vi "Update Front Panel.vi"() -> (3 "Battlefield":i32[][](array[numeric]))   [LabVIEW 2015, in "SB SubVIs.lvlib"]
uses:
  SB SubVIs.lvlib
  Globals.vi
  Globals (private).vi
  Square/Square.lvclass
  Endigit Library/Endigit.lvlib
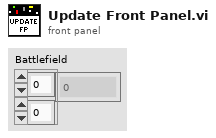
[diagram p1: front panel]
types:
  T1 = typedef "SB Type Defs.lvlib/Square Cluster.ctl" = cluster{"Attacked":bool, "Team":i32, "Next Turn":i32, "SEQ":refnum<queue>}
  T2 = typedef "SB Type Defs.lvlib/UI Refs.ctl" = cluster{"Battlefield":refnum<vi>, "Dashboard":refnum<vi>, "End Battle":refnum<vi>}
  T3 = cluster{"Color":u32, "Index":i32, "Status":string, "Stats":string}[]
  T4 = cluster{"Color":u32, "Index":i32, "Status":string, "Stats":string}
  T5 = cluster{"element":i32, "Config":cluster{"Color":u32, "Index":i32, "Status":string, "Stats":string}}
  T6 = cluster{"element":i32, "Config":cluster{"Color":u32, "Index":i32, "Status":string, "Stats":string}}[]
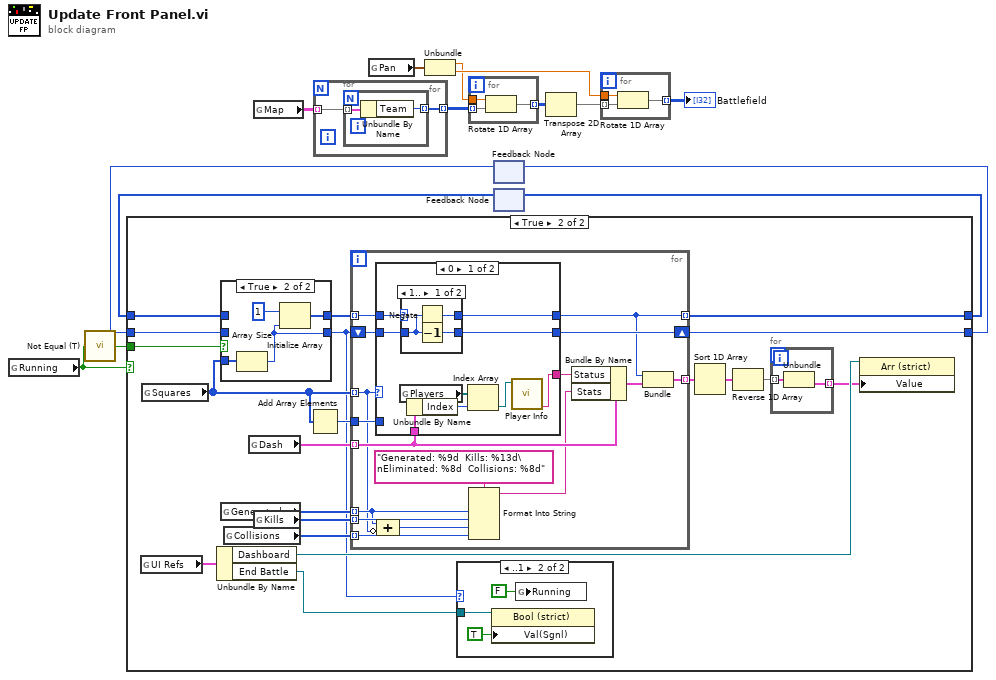
[diagram p0: block diagram]
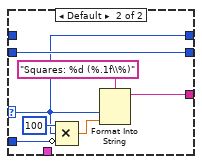
[diagram p6: hidden frame]
diagram:
  n1 = global read "Globals.vi" "Running"() -> (w7:bool)
  n2 = call "Not Equal (T).vi"("Variant"=w7) -> ("Changed"=w6:bool)
  n3 = global read "Globals.vi" "Map"() -> (w1:T1[][])
  n4 = for {
    tunnel: w1 -> [w16] mode=indexing
    tunnel: [w15] -> w9 mode=indexing
    n5 = for {
      tunnel: w16 -> [w18] mode=indexing
      tunnel: [w17] -> w15 mode=indexing
      n6 = Unbundle By Name(w18) -> ("Team"=w17:i32)
    }
  }
  n7 = global read "Globals.vi" "Pan"() -> (w12:cluster{"Horizontal":dbl, "Vertical":dbl})
  n8 = Unbundle(w12) -> ("Horizontal"=w13:dbl, "Vertical"=w14:dbl)
  n9 = for {
    tunnel: w9 -> [w21] mode=indexing
    tunnel: [w20] -> w10 mode=indexing
    tunnel: w13 -> [w19]
    n10 = Rotate 1D Array(1:w21, 2:w19) -> (0:w20:i32[])
  }
  n11 = feedback #1() -> (w4:i32)  [unwired: 1 in]
  n12 = feedback #2() -> (w2:i32[])  [unwired: 1 in]
  n13 = case shown="True" w7 {
    tunnel: w6 -> [_ w28]
    tunnel: [_ w26] -> w5
    tunnel: w4 -> [_ w25]
    tunnel: [_ w23] -> w3
    tunnel: w2 -> [_ w22]
    frame False {
    }
    frame True {
      n14 = global read "Globals.vi" "UI Refs"() -> (w40:T2)
      n15 = global read "Globals (private).vi" "Squares"() -> (w29:i32[])
      n16 = Unbundle By Name(w40) -> ("Dashboard"=w39:refnum<vi>, "End Battle"=w38:refnum<vi>)
      n17 = case shown="True" w28 {
        tunnel: w29 -> [_ w47]
        tunnel: [w43 w45] -> w27
        tunnel: w25 -> [w43 _]
        tunnel: [w42 w44] -> w24
        tunnel: w22 -> [w42 _]
        frame False {
        }
        frame True {
          n18 = Array Size(array=w47) -> (size(s)=w45:i32)
          n19 = Initialize Array(1, w45) -> (w44:i32[])
        }
      }
      n20 = global read "Globals (private).vi" "Generated"() -> (w37:i32[])
      n21 = global read "Globals (private).vi" "Collisions"() -> (w35:i32[])
      n22 = global read "Globals (private).vi" "Dash"() -> (w34:T3)
      n23 = global read "Globals (private).vi" "Kills"() -> (w36:i32[])
      n24 = Add Array Elements(numeric array=w29) -> (sum=w41:i32)
      n25 = for {
        tunnel: w34 -> [w66] mode=indexing
        tunnel: w29 -> [w60] mode=indexing
        tunnel: w41 -> [w67]
        tunnel: w37 -> [w61] mode=indexing
        tunnel: w36 -> [w63] mode=indexing
        tunnel: w35 -> [w62] mode=indexing
        tunnel: [w57] -> w33 mode=indexing
        tunnel: w24 -> [w54] mode=indexing
        tunnel: [w53] -> w23 mode=indexing
        shift-right: [w55] -> w26
        shift-left: w27 -> [w56]
        n26 = case shown="0" w60 {
          selector: w60 -> [_ w83]
          tunnel: [w77 w88] -> w68
          tunnel: w67 -> [_ w86]
          tunnel: w66 -> [w74 _]
          tunnel: w56 -> [w69 w84]
          tunnel: [w70 w84] -> w55
          tunnel: w54 -> [w72 _]
          tunnel: [w71 w83] -> w53
          frame 0 {
            n27 = global read "Globals (private).vi" "Players"() -> (w76:refnum<class "Square.lvclass">[])
            n28 = case shown="1.." w72 {
              selector: w72 -> [_ w82]
              tunnel: [w78 w82] -> w71
              tunnel: [w80 w81] -> w70
              tunnel: w69 -> [w79 w81]
              frame 1.. {
                n29 = Negate(x=w79) -> (-x=w78:i32)
                n30 = Decrement(x=w79) -> (x-1=w80:i32)
              }
              frame ..0 {
              }
            }
            n31 = Unbundle By Name(w74) -> ("Index"=w73:i32)
            n32 = Index Array(array=w76, index=w73) -> (element=w75:refnum<class "Square.lvclass">)
            n33 = call-dynamic "Player Info.vi"("Square in"=w75) -> ("Defeat Speech"=w77:string)  [unwired: 7 in, 3 out]
          }
          frame Default {
            n34 = Compound Arithmetic op=MULTIPLY(100 ("value"), w83, invert w86) -> (w87:dbl)
            n35 = Format Into String(format string="Squares: %d (%.1f\\%)", w83, w87) -> (resulting string=w88:string)  [unwired: 2 in, 1 out]
          }
        }
        n36 = Compound Arithmetic op=ADD(w61, invert w60) -> (w59:i32)
        n37 = Format Into String(format string="Generated: %9d  Kills: %13d\nEliminated: %8d  Collisions: %8d", w61, w63, w59, w62) -> (resulting string=w65:string)  [unwired: 2 in, 1 out]
        n38 = Bundle By Name(cluster=w66, "Status"=w68, "Stats"=w65) -> (w58:T4)
        n39 = Bundle("element"=w53, "Config"=w58) -> (w57:T5)  [unwired: 1 in]
      }
      n40 = case shown="..1" w27 {
        tunnel: w38 -> [_ w52]
        frame Default {
        }
        frame ..1 {
          n41 = property class="Bool (strict)"(reference=w52, "Val(Sgnl)"=TRUE ("Value (Signaling)")) -> ()  [unwired: 1 in, 2 out]
          n42 = global write "Globals.vi" "Running"(FALSE ("Running")) -> ()
        }
      }
      n43 = Sort 1D Array(array=w33) -> (sorted array=w32:T6)
      n44 = Reverse 1D Array(array=w32) -> (reversed array=w31:T6)
      n45 = for {
        tunnel: w31 -> [w49] mode=indexing
        tunnel: [w48] -> w30 mode=indexing
        n46 = Unbundle(w49) -> ("Config"=w48:T4)  [unwired: 1 out]
      }
      n47 = property class="Arr (strict)"(reference=w39, "Value"=w30) -> ()  [unwired: 1 in, 2 out]
    }
  }
  n48 = feedback-in #1(w5) -> ()
  n49 = feedback-in #2(w3) -> ()
  n50 = Transpose 2D Array(2D array=w10) -> (transposed array=w11:i32[][])
  n51 = for {
    tunnel: w11 -> [w92] mode=indexing
    tunnel: [w91] -> w8 mode=indexing
    tunnel: w14 -> [w90]
    n52 = Rotate 1D Array(1:w92, 2:w90) -> (0:w91:i32[])
  }
  "Battlefield" <- w8
